vi "FitTestCaitlyn.vi"() -> ()   [LabVIEW 2014]
uses:
  <vilib>/Utility/file.llb/Read From Spreadsheet File (DBL).vi
  <vilib>/Analysis/NI_AALPro.lvlib
panel:
  out "NMR":cluster{"Y":dbl[], "Y":dbl[]}[](graph)
  out "Fit Right Y":dbl[](array[numeric])
  out "Fit Left Y":dbl[](array[numeric])
  out "Fit Right":dbl[](array[numeric])
  out "Fit Left":dbl[](array[numeric])
  out "Fit Right":dbl[](array[numeric])
  out "Fit Left":dbl[](array[numeric])
  in  "Right wing":dbl
  in  "Left wing":dbl
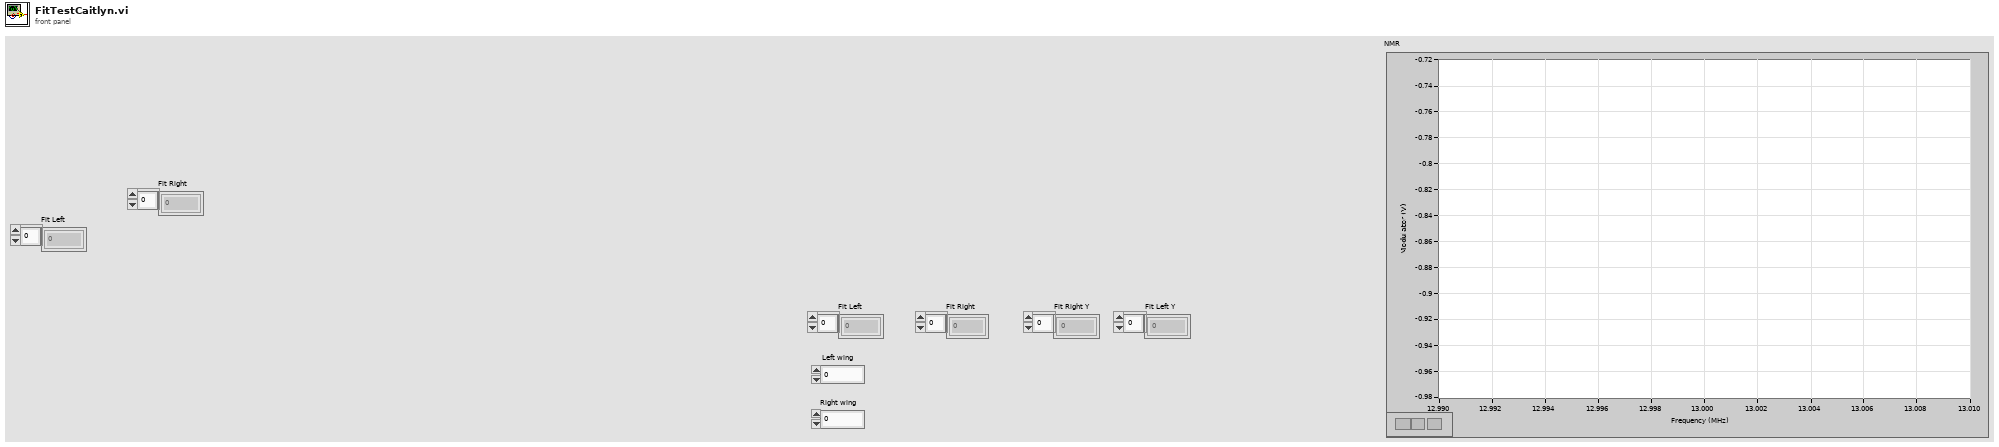
[diagram p1: front panel]
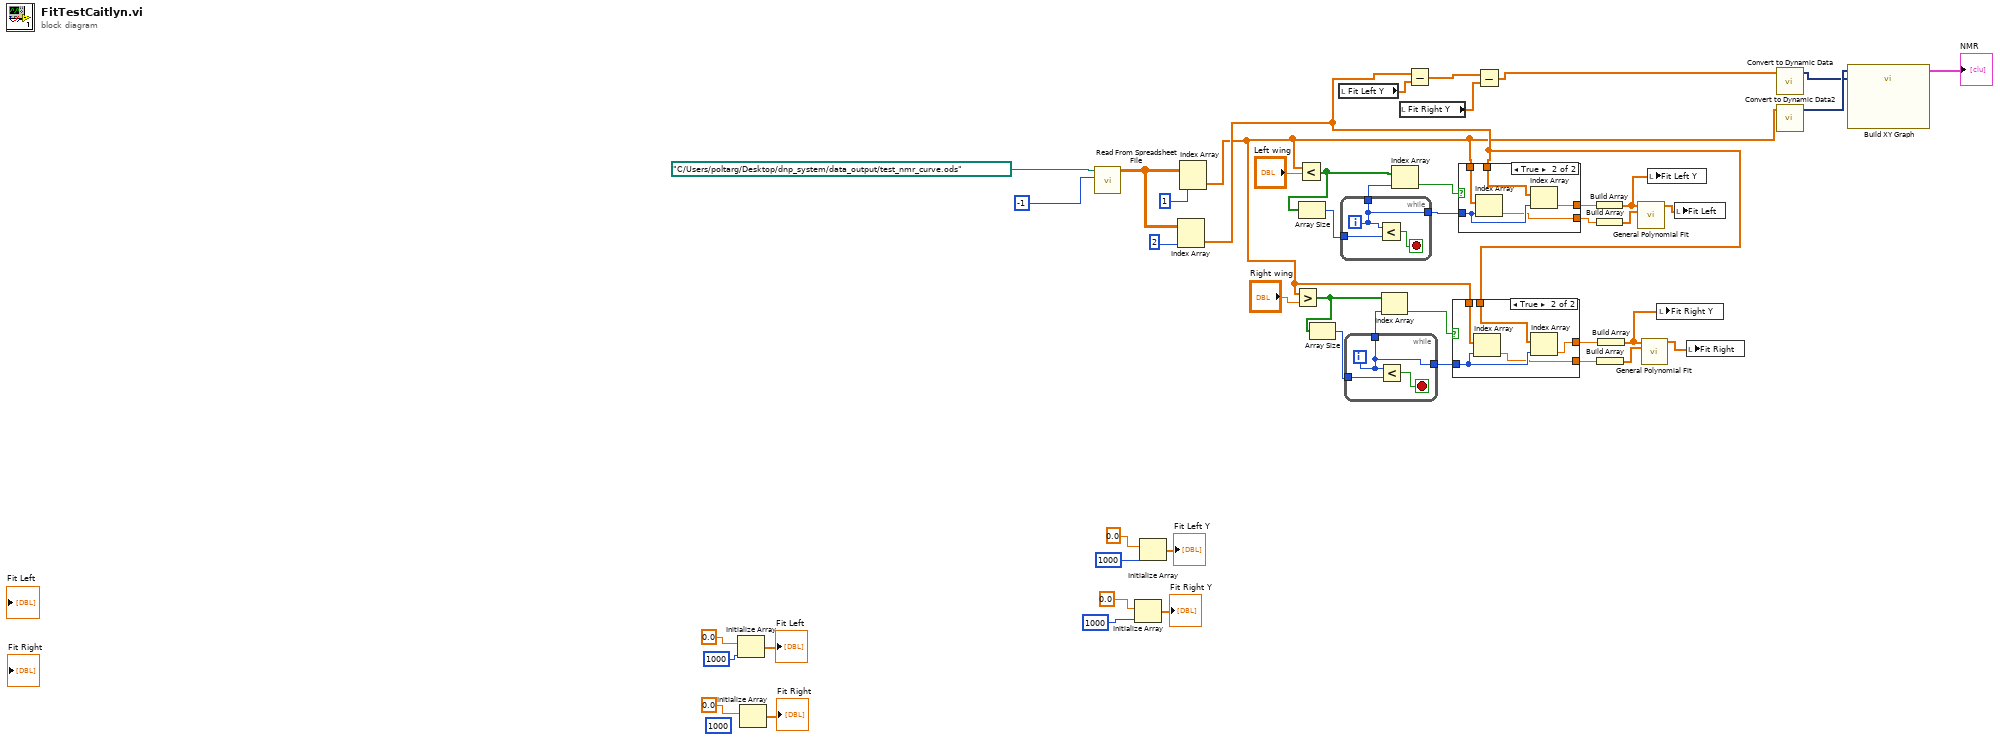
[diagram p0: block diagram]
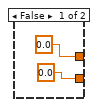
[diagram p2: hidden frame]
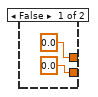
[diagram p3: hidden frame]
diagram:
  (unwired) 1000
  n1 = Initialize Array(0.0, 1000) -> (→"Fit Left":dbl[])
  n2 = Initialize Array(0.0) -> (→"Fit Right":dbl[])  [unwired: 1 in]
  n3 = call-poly <vilib>:"Read From Spreadsheet File.vi"("number of rows (all:-1)"=-1, "file path (dialog if empty)"=path "C:/Users/poltarg/Desktop/dnp_system/data_output/test_nmr_curve.ods") -> ("all rows"=w23:dbl[][])  [unwired: 5 in, 4 out]
  n4 = Initialize Array(0.0, 1000) -> (→"Fit Right Y":dbl[])
  n5 = Initialize Array(0.0, 1000) -> (→"Fit Left Y":dbl[])
  n6 = Index Array(array=w23, index (col)=2) -> (element=w20:dbl[])  [unwired: 1 in]
  n7 = Index Array(array=w23, index (col)=1) -> (element=w4:dbl[])  [unwired: 1 in]
  n8 = Greater?(x=w4, y="Right wing") -> (0:w37:bool[])
  n9 = Less?(x=w4, y="Left wing") -> (x < y?=w39:bool[])
  n10 = Array Size(array=w39) -> (size(s)=w44:i32)
  n11 = Array Size(array=w37) -> (size(s)=w36:i32)
  n12 = local read "Fit Left Y"() -> (w6:dbl[])
  n13 = while {
    tunnel: [w48] -> w45
    tunnel: w44 -> [w50]
    tunnel: [w48] -> w43
    i -> [w48]
    stop <- w49 stop-if-true
    n14 = Less?(x=w48, y=w50) -> (x < y?=w49:bool)
  }
  n15 = while {
    tunnel: w36 -> [w53]
    tunnel: [w51] -> w35
    tunnel: [w51] -> w33
    i -> [w51]
    stop <- w52 stop-if-true
    n16 = Less?(x=w51, y=w53) -> (x < y?=w52:bool)
  }
  n17 = Index Array(array=w37, index=w35) -> (element=w34:bool)
  n18 = Index Array(array=w39, index=w45) -> (element=w42:bool)
  n19 = local read "Fit Right Y"() -> (w5:dbl[])
  n20 = Subtract(x=w20, y=w6) -> (x-y=w47:dbl[])
  n21 = case shown="True" w34 {
    tunnel: w33 -> [_ w60]
    tunnel: w4 -> [_ w59]
    tunnel: w20 -> [_ w58]
    tunnel: [0.0 w57] -> w32
    tunnel: [0.0 w56] -> w31
    frame False {
    }
    frame True {
      n22 = Index Array(array=w59, index=w60) -> (element=w56:dbl)
      n23 = Index Array(array=w58, index=w60) -> (element=w57:dbl)
    }
  }
  n24 = case shown="True" w42 {
    tunnel: w4 -> [_ w67]
    tunnel: w20 -> [_ w66]
    tunnel: w43 -> [_ w65]
    tunnel: [0.0 w64] -> w41
    tunnel: [0.0 w63] -> w40
    frame False {
    }
    frame True {
      n25 = Index Array(array=w67, index=w65) -> (element=w64:dbl)
      n26 = Index Array(array=w66, index=w65) -> (element=w63:dbl)
    }
  }
  n27 = Subtract(x=w47, y=w5) -> (x-y=w26:dbl[])
  n28 = Build Array(w40) -> (w7:dbl[])
  n29 = Build Array(w41) -> (w28:dbl[])
  n30 = Build Array(w31) -> (w30:dbl[])
  n31 = Build Array(w32) -> (w8:dbl[])
  n32 = call <vilib>:"General Polynomial Fit.vi"("Y"=w7, "X"=w28) -> ("Best Polynomial Fit"=w27:dbl[])  [unwired: 10 in, 3 out]
  n33 = call <vilib>:"General Polynomial Fit.vi"("Y"=w8, "X"=w30) -> ("Best Polynomial Fit"=w29:dbl[])  [unwired: 10 in, 3 out]
  n34 = local write "Fit Left Y"(w7) -> ()
  n35 = local write "Fit Right Y"(w8) -> ()
  n36 = local write "Fit Left"(w27) -> ()
  n37 = local write "Fit Right"(w29) -> ()
  n38 = call "Convert to Dynamic Data"("Array"=w26) -> ("Dynamic Data Type"=w2:dynamicdata)  [unwired: 3 in]
  n39 = call "Convert to Dynamic Data2"("Array"=w4) -> ("Dynamic Data Type"=w3:dynamicdata)  [unwired: 3 in]
  n40 = call "Build XY Graph"("Y Input"=w2, "X Input"=w3) -> ("XY Graph"=→"NMR":cluster{"Y":dbl[], "Y":dbl[]}[])  [unwired: 8 in, 1 out]
